vi "Set Intake autonomous.vi"(8 "error in (no error)":errorcluster) -> (0 "error out":errorcluster)   [LabVIEW 2013]
uses:
  InTake/InTake Global Data.vi
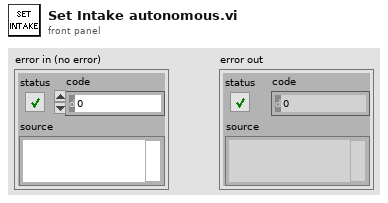
[diagram p1: front panel]
types:
  T1 = cluster{"TakeBall":dbl, "UpperClaw":dbl, "MS":bool, "Upper claw max":bool, "Upper claw min":bool, "Angle":dbl}
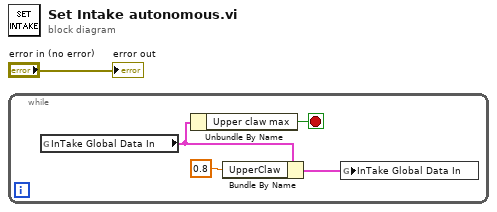
[diagram p0: block diagram]
diagram:
  n1 = while {
    stop <- w2 stop-if-true
    n2 = global read "InTake Global Data.vi" "InTake Global Data In"() -> (w3:T1)
    n3 = Unbundle By Name(w3) -> ("Upper claw max"=w2:bool)
    n4 = Bundle By Name(cluster=w3, "UpperClaw"=0.8 ("Output")) -> (w5:T1)
    n5 = global write "InTake Global Data.vi" "InTake Global Data In"(w5) -> ()
  }
  "error out" <- "error in (no error)"
